vi "Contrast Keller.vi"(8 "error in":errorcluster, 10 "histogram bins":sgl[](array[numeric]), 11 "histogram counts":sgl[](array[numeric])) -> (0 "error out":errorcluster, 3 "Contrast":sgl)   [LabVIEW 2012, in "MeritFactor.lvclass"]
uses:
  MeritFactor.lvclass
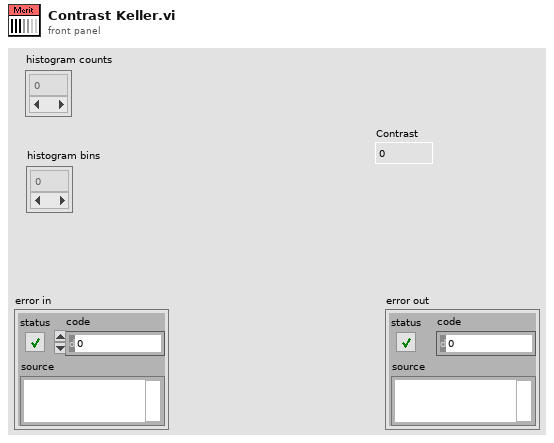
[diagram p1: front panel]
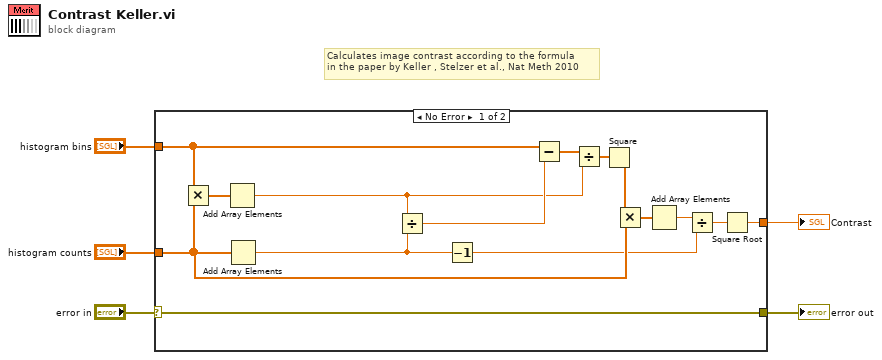
[diagram p0: block diagram]
diagram:
  # "Calculates image contrast according to the formula\nin the paper by Keller , Stelzer et al., Nat Meth 2010"
  n1 = case shown="No Error" "error in" {
    selector: "error in" -> [w6 w21]
    tunnel: "histogram counts" -> [w13 _]
    tunnel: "histogram bins" -> [w19 _]
    tunnel: [w7 _] -> w2
    tunnel: [w6 w21] -> w1
    frame No Error {
      n2 = Multiply(x=w19, y=w13) -> (x*y=w20:sgl[])
      n3 = Add Array Elements(numeric array=w20) -> (sum=w16:sgl)
      n4 = Add Array Elements(numeric array=w13) -> (sum=w11:sgl)
      n5 = Divide(x=w16, y=w11) -> (x/y=w18:sgl)
      n6 = Decrement(x=w11) -> (x-1=w9:sgl)
      n7 = Subtract(x=w19, y=w18) -> (x-y=w17:sgl[])
      n8 = Divide(x=w17, y=w16) -> (x/y=w15:sgl[])
      n9 = Square(x=w15) -> (x^2=w14:sgl[])
      n10 = Multiply(x=w14, y=w13) -> (x*y=w12:sgl[])
      n11 = Add Array Elements(numeric array=w12) -> (sum=w10:sgl)
      n12 = Divide(x=w10, y=w9) -> (x/y=w8:sgl)
      n13 = Square Root(x=w8) -> (sqrt(x)=w7:sgl)
    }
    frame Error {
    }
  }
  "error out" <- w1
  "Contrast" <- w2
